vi "ULx Write (Counter 1D Time NChan 1Samp).vi"(0 "task in":refnum<k24>, 1 "auto start":bool=TRUE, 7 "data":cluster{"high time":dbl, "low time":dbl}[](array[cluster]), 9 "timeout":dbl=10.0 format="%_4g", 11 "error in":errorcluster) -> (4 "task out":refnum<k24>, 10 "number of samples written per channel":u32, 15 "error out":errorcluster)   [LabVIEW 2020]
doc: "Writes a new pulse high time and low time to each channel in a counter output task that contains one or more channels."
uses:
  C:/Users/William/Documents/LV 2020 builds/LeaktestDAQ/Source-v33/ULx_LV.dll
  ULx_LV.dll
panel:
  # "channel"
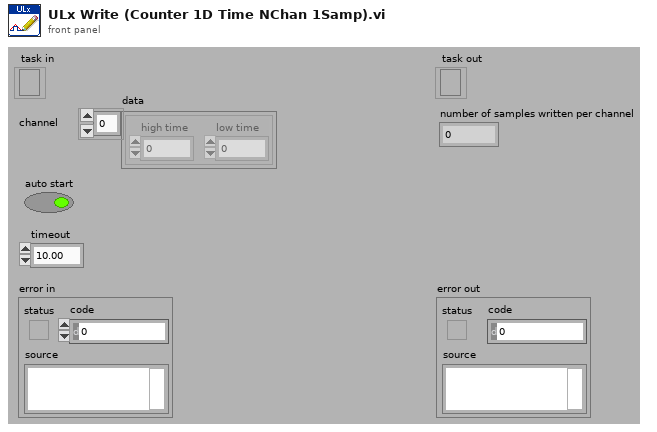
[diagram p1: front panel]
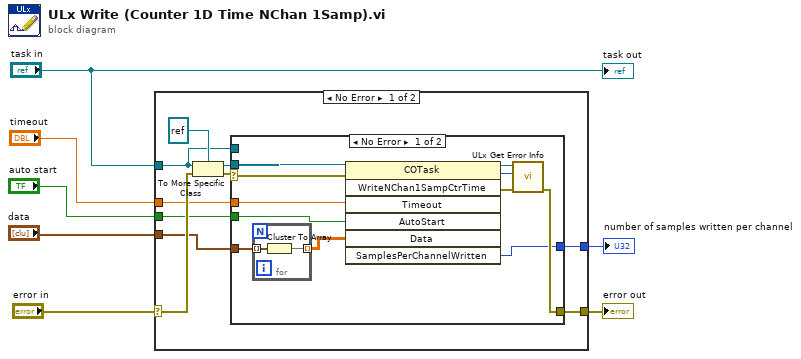
[diagram p0: block diagram]
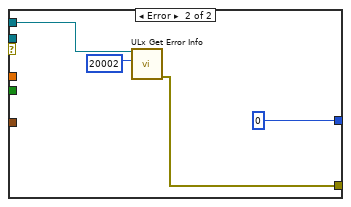
[diagram p2: hidden frame]
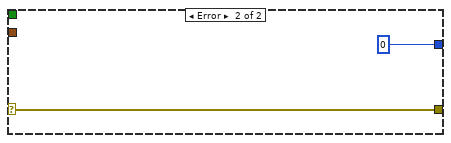
[diagram p3: hidden frame]
diagram:
  n1 = case shown="No Error" "error in" {
    selector: "error in" -> [w17 w36]
    tunnel: "task in" -> [w11 _]
    tunnel: "timeout" -> [w13 _]
    tunnel: [w12 w36] -> w5
    tunnel: "auto start" -> [w10 _]
    tunnel: [w9 0 ("SamplesPerChannelWritten")] -> w2
    tunnel: "data" -> [w8 _]
    frame No Error {
      n2 = To More Specific Class(target class=refnum<k24> refnum, reference=w11, error in=w17) -> (specific class reference=w14:refnum<k24>, error out=w15:errorcluster)
      n3 = case shown="No Error" w15 {
        selector: w15 -> [w27 _]
        tunnel: w14 -> [w28 _]
        tunnel: w13 -> [w21 _]
        tunnel: [w24 w33] -> w12
        tunnel: w11 -> [_ w32]
        tunnel: w10 -> [w20 _]
        tunnel: [w22 0 ("SamplesPerChannelWritten")] -> w9
        tunnel: w8 -> [w19 _]
        frame No Error {
          n4 = for {
            tunnel: w19 -> [w30] mode=indexing
            tunnel: [w29] -> w18 mode=indexing
            n5 = Cluster To Array(cluster=w30) -> (array=w29:dbl[])
          }
          n6 = invoke class="COTask" method="WriteNChan1SampCtrTime"(reference=w28, error in=w27, "Timeout"=w21, "AutoStart"=w20, "Data"=w18) -> (reference out=w25:refnum<k24>, error out=w26:errorcluster, "WriteNChan1SampCtrTime"=w23:i32, "SamplesPerChannelWritten"=w22:u32)  [unwired: 2 in, 3 out]
          n7 = call "ULx Get Error Info.vi"("error in"=w26, "ErrorCode"=w23, "task in"=w25) -> ("error out"=w24:errorcluster)  [unwired: 8 in]
        }
        frame Error {
          n8 = call "ULx Get Error Info.vi"("ErrorCode"=20002, "task in"=w32) -> ("error out"=w33:errorcluster)  [unwired: 9 in]
        }
      }
    }
    frame Error {
    }
  }
  "error out" <- w5
  "number of samples written per channel" <- w2
  "task out" <- "task in"
